vi "testUintAdd.vi"(8 "error in (no error)":errorcluster, 11 "TestCase in":refnum<class "UnitTestUintClass.lvclass">) -> (0 "error out":errorcluster, 3 "TestCase out":refnum<class "UnitTestUintClass.lvclass">)   [LabVIEW 2011, in "UnitTestUintClass.lvclass"]
uses:
  UnitTestUintClass.lvclass
  UnitTestUintClass.lvclass/UnitTestUintClass.ctl
  <vilib>/addons/_JKI Toolkits/VI Tester/TestCase.llb/TestCase.lvclass
  UintClass/UintClass.lvclass
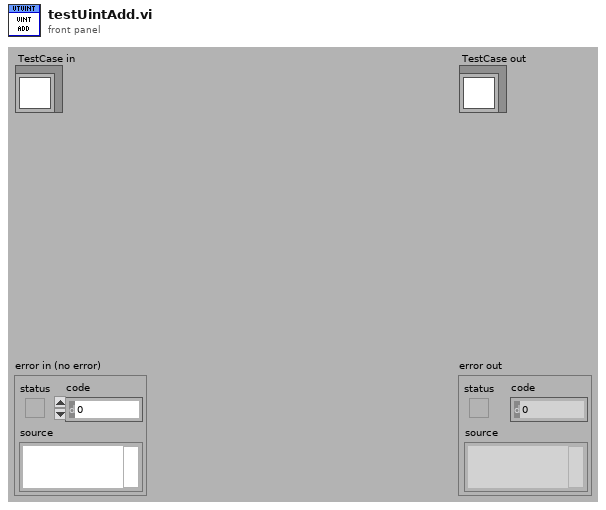
[diagram p1: front panel]
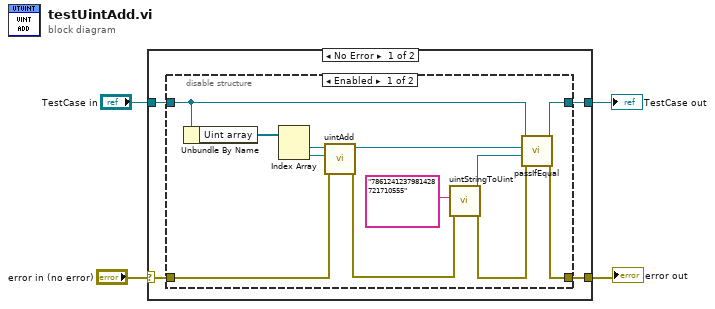
[diagram p0: block diagram]
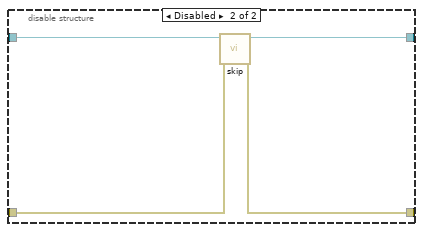
[diagram p2: hidden frame]
diagram:
  n1 = case shown="No Error" "error in (no error)" {
    selector: "error in (no error)" -> [w6 w26]
    tunnel: [w5 w26] -> w3
    tunnel: [w7 w25] -> w1
    tunnel: "TestCase in" -> [w8 w25]
    frame No Error {
      n2 = disable-structure shown="Enabled" {
        disable-tunnel: w8 -> [w18 w24]
        disable-tunnel: [w20 w21] -> w7
        disable-tunnel: w6 -> [w11 w23]
        disable-tunnel: [w19 w22] -> w5
        frame Enabled {
          n3 = Unbundle By Name(w18) -> ("Uint array"=w17:refnum<class "UintClass.lvclass">[])
          n4 = Index Array(array=w17) -> (element #1=w16:refnum<class "UintClass.lvclass">, element #2=w15:refnum<class "UintClass.lvclass">)  [unwired: 2 in]
          n5 = call "uintAdd.vi"("Error in (no error)"=w11, "Uint2 in"=w15, "Uint1 in"=w16) -> ("Error out"=w12:errorcluster, "Uint1 + Uint2"=w14:refnum<class "UintClass.lvclass">)  [unwired: 6 in, 1 out]
          n6 = call "uintStringToUint.vi"("Error in (no error)"=w12, "String in"="7861241237981428721710555") -> ("Error out"=w10:errorcluster, "Uint out"=w13:refnum<class "UintClass.lvclass">)  [unwired: 8 in]
          n7 = call-dynamic "passIfEqual.vi"("error in (no error)"=w10, "y"=w13, "x"=w14, "TestCase in"=w18) -> ("error out"=w19:errorcluster, "TestCase out"=w20:refnum<class "UnitTestUintClass.lvclass">)  [unwired: 6 in]
        }
        frame Disabled {
          n8 = call <vilib>:"skip.vi"("error in (no error)"=w23, "TestCase in"=w24) -> ("error out"=w22:errorcluster, "TestCase out"=w21:refnum<class "UnitTestUintClass.lvclass">)  [unwired: 8 in]
        }
      }
    }
    frame Error {
    }
  }
  "error out" <- w3
  "TestCase out" <- w1
